vi "lxw name to col 2.vi"(8 "error in (no error)":errorcluster, 11 "col_str":string) -> (0 "error out":errorcluster, 3 "function return":u16)   [LabVIEW 8.6]
doc: "uint16_t lxw_name_to_col_2(const char *col_str);"
uses:
  pending_lvxlsxwriter/xlsxwriter.dll
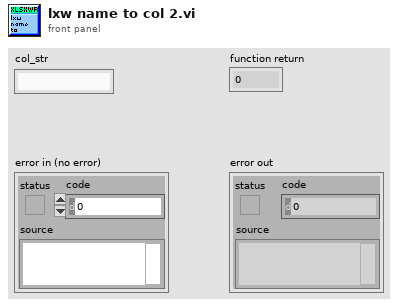
[diagram p1: front panel]
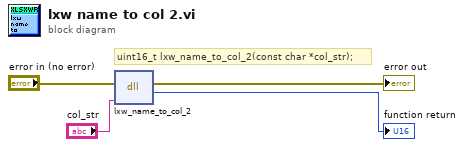
[diagram p0: block diagram]
diagram:
  # "uint16_t lxw_name_to_col_2(const char *col_str);"
  n1 = dll-call lib="C:/Users/WDAGUtilityAccount/Desktop/pending_lvxlsxwriter/xlsxwriter.*" fn="lxw_name_to_col_2"(error in="error in (no error)", "col_str"="col_str") -> (error out=→"error out":errorcluster, →"function return":u16)  [unwired: 3 in, 1 out]
